vi "UDP Multicast Sender Test.vi"() -> ()   [LabVIEW 2020]
uses:
  <vilib>/Utility/tcp.llb/UDP Multicast Read-Write Open.vi
panel:
  out "data out":string
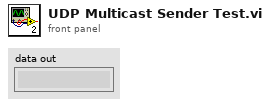
[diagram p1: front panel]
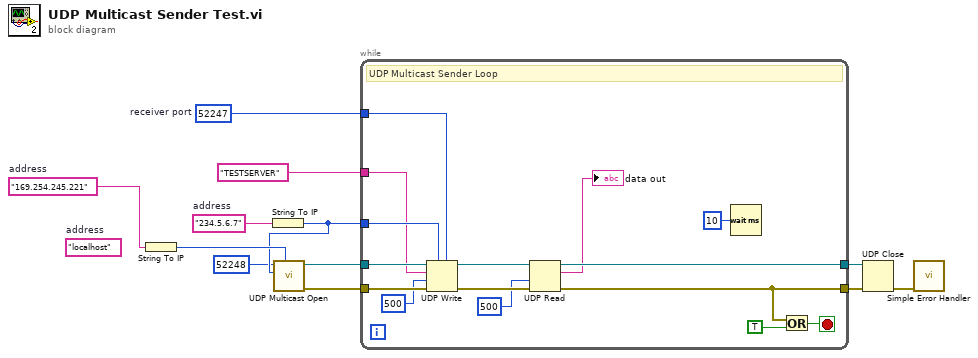
[diagram p0: block diagram]
diagram:
  w3 = "169.254.245.221"  # address
  (unwired) "localhost"  # address
  w6 = u16 52247  # receiver port
  w10 = "234.5.6.7"  # address
  n1 = String To IP(1:w3) -> (0:w4:u32)
  n2 = String To IP(1:w10) -> (0:w2:u32)
  n3 = call-poly <vilib>:"UDP Multicast Open.vi"("net address"=w4, "multicast addr"=w2, "port"=u16 52248) -> ("error out"=w7:errorcluster, "connection ID"=w8:refnum<k16>)  [unwired: 6 in, 1 out]
  n4 = while {
    tunnel: [w16] -> w11
    tunnel: w8 -> [w27]
    tunnel: w7 -> [w26]
    tunnel: [w17] -> w12
    tunnel: w2 -> [w24]
    tunnel: w6 -> [w22]
    tunnel: "TESTSERVER" -> [w21]
    stop <- w25 stop-if-true
    # "UDP Multicast Sender Loop"
    n5 = UDP Write(address=w24, port or service name=w22, connection ID=w27, data in=w21, 8:w26, 9:500 ("timeout ms (25000)")) -> (error out=w18:errorcluster, 3:w19:refnum<k16>)
    n6 = UDP Read(connection ID=w19, timeout ms (25000)=500, 8:w18) -> (data out=→"data out":string, error out=w16:errorcluster, 3:w17:refnum<k16>)  [unwired: 3 out]
    n7 = Wait (ms)(milliseconds to wait=u32 10) -> ()  [unwired: 1 out]
    n8 = Or(x=w16, y=TRUE) -> (x .or. y?=w25:bool)
  }
  n9 = UDP Close(connection ID=w12, 8:w11) -> (error out=w9:errorcluster)  [unwired: 1 out]
  n10 = call <vilib>:"Simple Error Handler.vi"("error in (no error)"=w9) -> ()  [unwired: 4 in, 5 out]
